vi "init.vi"(0 "Constant Analog Output Voltage Test in":refnum<class "Constant Analog Output Voltage Test.lvclass">, 1 "DAQ Channel":refnum<k21>, 2 "Expected Value":dbl format="%.3f", 3 "Tolerance":dbl format="%.3f", 4 "Samples To Average":i32, 5 "error in (no error)":errorcluster, 6 "MustPass?":bool, 7 "Log":refnum<class "ITestLog.lvclass">, 8 "Test Scenario":T1, 10 "Signal Name":string) -> (14 "Constant Analog Output Voltage Test  out":refnum<class "Constant Analog Output Voltage Test.lvclass">, 19 "error out":errorcluster)   [LabVIEW 2015, in "Constant Analog Output Voltage Test.lvclass"]
uses:
  Constant Analog Output Voltage Test.lvclass
  Model/TestLog/ITestLog/ITestLog.lvclass
  Typedefs/TestScenarioTypes.ctl
  Constant Analog Output Voltage Test.lvclass/Constant Analog Output Voltage Test.ctl
  Typedefs/ILCBTTypedefs.lvlib
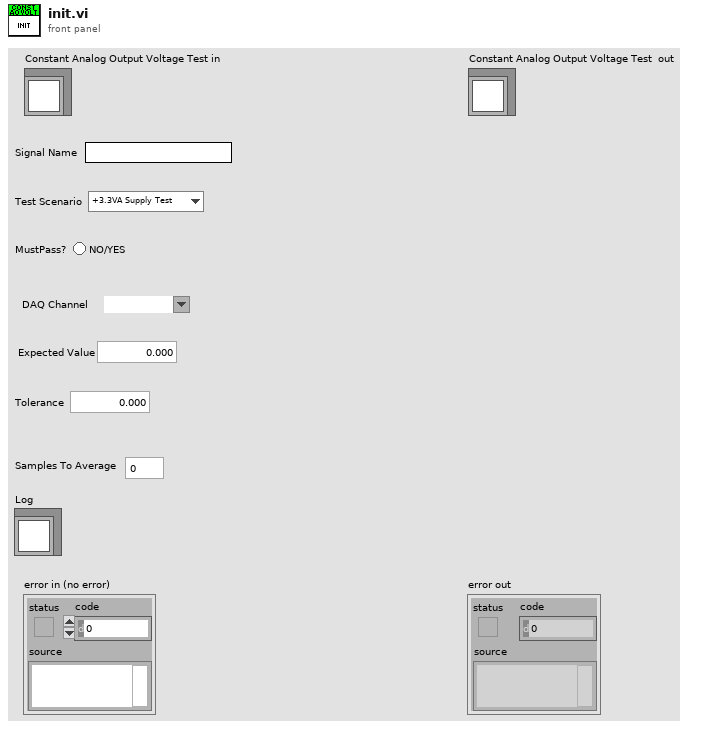
[diagram p1: front panel]
types:
  T1 = typedef "ILCBTTypedefs.lvlib/TestScenarioTypes.ctl" = enum16{"+3.3VA Supply Test", "+3.3VD Supply Test", "+5VA Supply Test", "+5VD Supply Test", "Unique ID Test", "TEDS Status Test", "LIMSW1_TTL Low Test", "LIMSW1_TTL High Test", "LIMSW2_TTL Low Test", "LIMSW2_TTL High Test", "Tachometer Test", "SSR_TTL Low Test", "SSR_TTL High Test", "SM_CW Low Test", "SM_CW High Test", "SM_CCW Low Test", "SM_CCW High Test", "SM_GPI Low Test", "SM_GPI High Test", "CW Motion Without Limit Test", "CW Motion With Limit Test", "CW Motion With Limit Interruption Test", "CW Motion on CCW Limit Test", "CCW Motion Without Limit Test", "CCW Motion With Limit Test", "CCW Motion With Limit Interruption Test", "CCW Motion on CW Limit Test", "RS232-TXD Low Test", "RS232-TXD High Test", "RS232-RTS Low Test", "RS232-RTS High Test", "RS232-RXD Low Test", "RS232-RXD High Test", "RS232-CTS Low Test", "RS232-CTS High Test", "Out_SS Low Test", "Out_SS High Test", "Out_SDI Low Test", "Out_SDI High Test", "Out_SCLK Low Test", "Out_SCLK High Test", "Reset Low Test", "Reset High Test", "1 Channel ADC Test", "3 Channel ADC Test", "5 Channel ADC Test", "Vref Test", "ROT Test", "DAC1 Test", "DAC2 Test", "DAC3 Test", "DAC4 Test", "BIAS Test", "EXC1 Test", "EXC2 Test", "EXC3 Test", "EXC4 Test"}
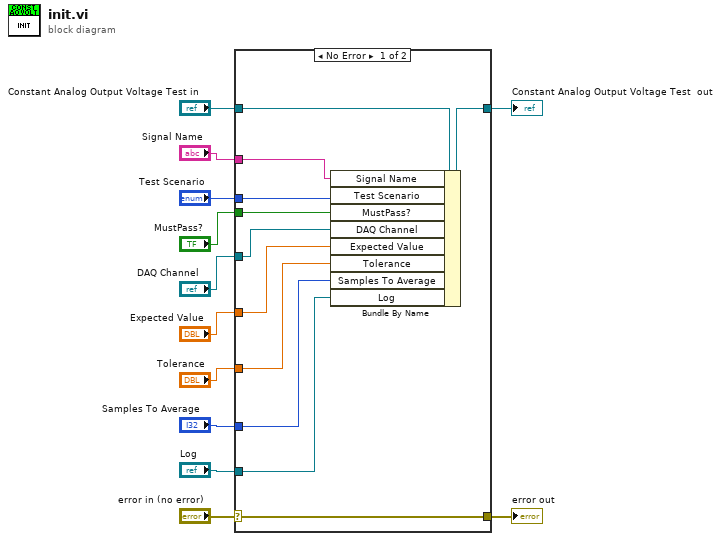
[diagram p0: block diagram]
diagram:
  n1 = case shown="No Error" "error in (no error)" {
    selector: "error in (no error)" -> [w23 w25]
    tunnel: [w23 w25] -> w11
    tunnel: [w21 w24] -> w9
    tunnel: "Constant Analog Output Voltage Test in" -> [w22 w24]
    tunnel: "DAQ Channel" -> [w20 _]
    tunnel: "Expected Value" -> [w19 _]
    tunnel: "Tolerance" -> [w18 _]
    tunnel: "Samples To Average" -> [w17 _]
    tunnel: "Log" -> [w16 _]
    tunnel: "Signal Name" -> [w14 _]
    tunnel: "Test Scenario" -> [w13 _]
    tunnel: "MustPass?" -> [w15 _]
    frame No Error {
      n2 = Bundle By Name(cluster=w22, "Signal Name"=w14, "Test Scenario"=w13, "MustPass?"=w15, "DAQ Channel"=w20, "Expected Value"=w19, "Tolerance"=w18, "Samples To Average"=w17, "Log"=w16) -> (w21:refnum<class "Constant Analog Output Voltage Test.lvclass">)
    }
    frame Error {
    }
  }
  "error out" <- w11
  "Constant Analog Output Voltage Test  out" <- w9
